vi "Update Table by String Array.vi"(4 "PK value":string, 6 "PK column":string, 7 "data":string[](array[string]), 8 "error in (no error)":errorcluster, 9 "columns":string[](array[string]), 10 "table":string, 11 "ADODB in":refnum<class "ADODB.lvclass">) -> (0 "error out":errorcluster, 3 "ADODB out":refnum<class "ADODB.lvclass">)   [LabVIEW 2020, in "ADODB.lvlib" / "ADODB.lvclass"]
uses:
  ADODB.lvclass
  ADODB.lvclass/ADODB.ctl
  <vilib>/addons/database/Connection.llb/Conn Execute.vi
  <vilib>/addons/database/Recordset.llb/Rec Destroy - Connection.vi
  DBMS Specific/DBMS Specific.lvclass
  <vilib>/addons/database/NI_Database_API.lvlib
panel:
  # "This VI does not correct for \"Data\" and \"Pk values\"\nstring formatting. I.e., most DBMS require non-numeric \nvalues to have single quotes around them, 'value'"
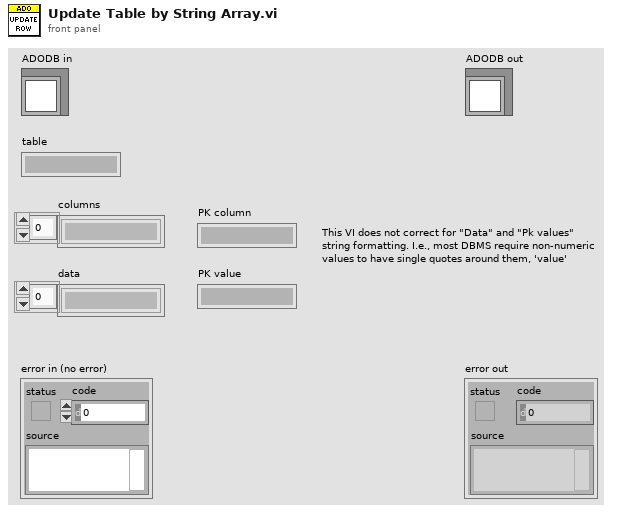
[diagram p1: front panel]
types:
  T1 = typedef "NI_Database_API.lvlib/Conn ObjectReference.ctl" = refnum<k1>
  T2 = typedef "NI_Database_API.lvlib/Rec ObjectReference.ctl" = refnum<k1>
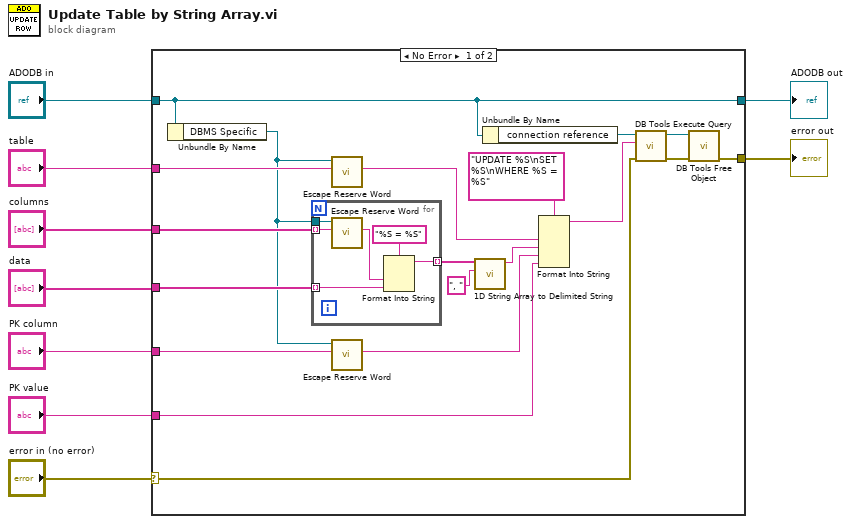
[diagram p0: block diagram]
diagram:
  n1 = case shown="No Error" "error in (no error)" {
    selector: "error in (no error)" -> [w14 w36]
    tunnel: "columns" -> [w20 _]
    tunnel: "data" -> [w18 _]
    tunnel: [w24 w36] -> w7
    tunnel: "ADODB in" -> [w23 w35]
    tunnel: [w23 w35] -> w8
    tunnel: "table" -> [w22 _]
    tunnel: "PK column" -> [w12 _]
    tunnel: "PK value" -> [w10 _]
    frame No Error {
      n2 = Unbundle By Name(w23) -> ("DBMS Specific"=w13:refnum<class "DBMS Specific.lvclass">)
      n3 = for {
        tunnel: w13 -> [w29]
        tunnel: w20 -> [w34] mode=indexing
        tunnel: w18 -> [w31] mode=indexing
        tunnel: [w30] -> w16 mode=indexing
        n4 = call-dynamic "Escape Reserve Word.vi"("Input Name"=w34, "DBMS Specific in"=w29) -> ("Escaped Name"=w32:string)  [unwired: 7 in, 2 out]
        n5 = Format Into String(format string="%S = %S", w32, w31) -> (resulting string=w30:string)  [unwired: 2 in, 1 out]
      }
      n6 = call-dynamic "Escape Reserve Word.vi"("Input Name"=w22, "DBMS Specific in"=w13) -> ("Escaped Name"=w21:string)  [unwired: 7 in, 2 out]
      n7 = call-dynamic "Escape Reserve Word.vi"("Input Name"=w12, "DBMS Specific in"=w13) -> ("Escaped Name"=w11:string)  [unwired: 7 in, 2 out]
      n8 = call <vilib>:"1D String Array to Delimited String.vi"("delimiter"=", ", "string array"=w16) -> ("delimited string"=w15:string)  [unwired: 9 in]
      n9 = Unbundle By Name(w23) -> ("connection reference"=w27:T1)
      n10 = Format Into String(format string="UPDATE %S\nSET %S\nWHERE %S = %S", w21, w15, w11, w10) -> (resulting string=w28:string)  [unwired: 2 in, 1 out]
      n11 = call-poly <vilib>:"DB Tools Execute Query.vi"("error in (no error)"=w14, "SQL query"=w28, "connection reference"=w27) -> ("error out"=w25:errorcluster, "recordset reference"=w26:T2)  [unwired: 5 in]
      n12 = call-poly <vilib>:"DB Tools Free Object.vi"("error in (no error)"=w25, "recordset reference"=w26) -> ("error out"=w24:errorcluster)  [unwired: 8 in, 1 out]
    }
    frame Error {
    }
  }
  "error out" <- w7
  "ADODB out" <- w8
